vi "Stop Collection.vi"(8 "error in (no error)":errorcluster, 11 "Modeli in":refnum<class "Modeli.lvclass">) -> (0 "error out":errorcluster, 3 "Modeli out":refnum<class "Modeli.lvclass">)   [LabVIEW 2018, in "Modeli.lvlib" / "Modeli.lvclass"]
uses:
  Modeli.lvclass
  Projects/PRJ-Quasar Listening/Quasar Listening/x64/Release/Quasar Listening.dll
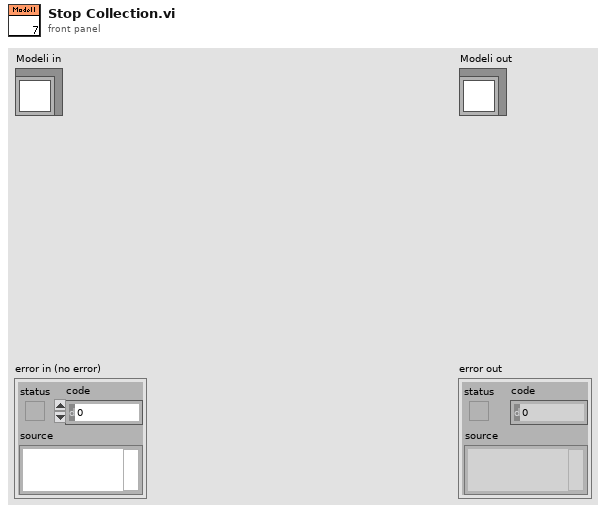
[diagram p1: front panel]
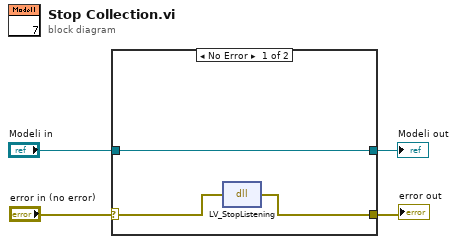
[diagram p0: block diagram]
diagram:
  n1 = case shown="No Error" "error in (no error)" {
    selector: "error in (no error)" -> [w7 w8]
    tunnel: [w6 w8] -> w3
    tunnel: "Modeli in" -> [w5 w9]
    tunnel: [w5 w9] -> w1
    frame No Error {
      n2 = dll-call lib="C:/Projects/PRJ-Quasar Listening/Quasar Listening/x64/Release/Quasar Listening.dll" fn="LV_StopListening"(error in=w7) -> (error out=w6:errorcluster)  [unwired: 3 in, 1 out]
    }
    frame Error {
    }
  }
  "error out" <- w3
  "Modeli out" <- w1
